vi "COMI ENC Load.vi"(9 "Count":i32, 10 "ch":i32, 11 "hDevice":u32) -> (3 "hDevice out":u32)   [LabVIEW 2017, in "Comidll.lvlib"]
doc: "void (COMI_ENC_Load) (HANDLE hDevice, int ch, long Count);"
uses:
  <userlib>/Comidll/Comidll.lvlib
  <userlib>/Comidll/Comidll.dll
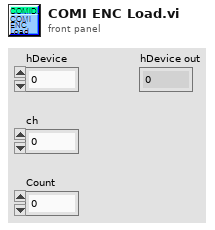
[diagram p1: front panel]
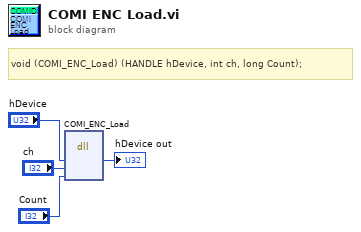
[diagram p0: block diagram]
diagram:
  # "void\t(COMI_ENC_Load) (HANDLE hDevice, int ch, long Count);"
  n1 = dll-call lib="C:/Program Files/National Instruments/LabVIEW 2017/user.lib/Comidll/Comidll.*" fn="COMI_ENC_Load"("hDevice"="hDevice", "ch"="ch", "Count"="Count") -> ("hDevice"=→"hDevice out":u32)  [unwired: 6 in, 2 out]
